vi "init.vi"(0 "EXC1Test in":refnum<class "EXC1Test.lvclass">, 1 "Tolerance":dbl[unit], 5 "Log":refnum<class "ITestLog.lvclass">, 7 "DAQ Channel To Read":refnum<k21>, 9 "Expected Value":dbl[unit], 11 "error in (no error)":errorcluster, 12 "Samples To Read":dbl) -> (4 "EXC1Test out":refnum<class "EXC1Test.lvclass">, 15 "error out":errorcluster)   [LabVIEW 2015, in "EXC1Test.lvclass"]
uses:
  EXC1Test.lvclass
  Model/TestLog/ITestLog/ITestLog.lvclass
  EXC1Test.lvclass/EXC1Test.ctl
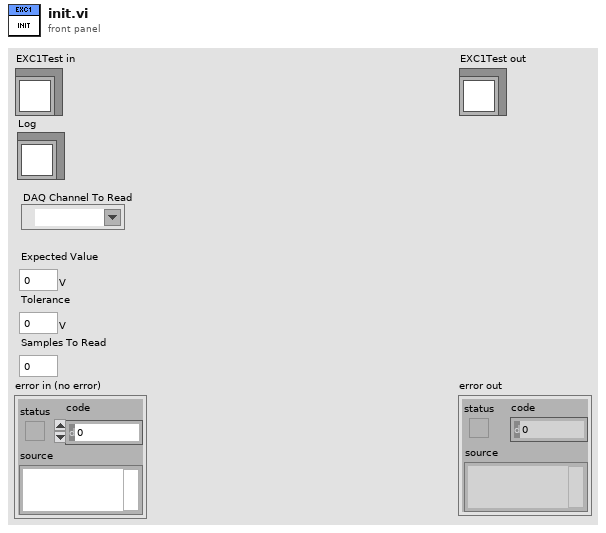
[diagram p1: front panel]
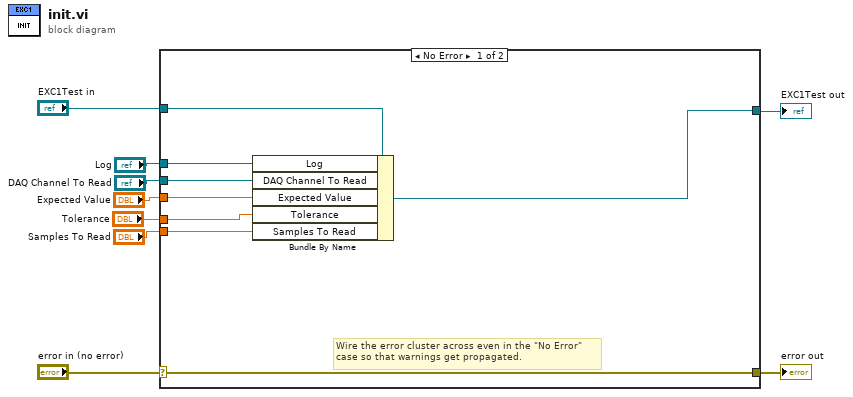
[diagram p0: block diagram]
diagram:
  n1 = case shown="No Error" "error in (no error)" {
    selector: "error in (no error)" -> [w17 w19]
    tunnel: [w17 w19] -> w8
    tunnel: [w10 w18] -> w6
    tunnel: "EXC1Test in" -> [w16 w18]
    tunnel: "Log" -> [w15 _]
    tunnel: "DAQ Channel To Read" -> [w14 _]
    tunnel: "Expected Value" -> [w13 _]
    tunnel: "Tolerance" -> [w12 _]
    tunnel: "Samples To Read" -> [w11 _]
    frame No Error {
      # "Wire the error cluster across even in the \"No Error\"\ncase so that warnings get propagated."
      n2 = Bundle By Name(cluster=w16, "Log"=w15, "DAQ Channel To Read"=w14, "Expected Value"=w13, "Tolerance"=w12, "Samples To Read"=w11) -> (w10:refnum<class "EXC1Test.lvclass">)
    }
    frame Error {
    }
  }
  "error out" <- w8
  "EXC1Test out" <- w6
